vi "RT Main.vi"() -> ()   [LabVIEW 2025]
doc: "The myRIO Custom FPGA Project template acquires button data from the onboard button and displays the button value on a Boolean indicator. The SYS.RDY indicator shows the FPGA status."
uses:
  <vilib>/rvi/interface/nirviOpenFPGA/nirviOpenFPGA.xnode
  <vilib>/rvi/interface/nirviCloseFPGA/nirviCloseFPGA.xnode
  <vilib>/rvi/interface/nirviMethod/nirviMethod.xnode
  <vilib>/FPGAPlugInAG/Dynamic/niLvFpga_Run_Dynamic.vi
  SoC IP Library/SoC IP Library.lvlib
  SoC IP Library/Controls/Image Size.ctl
  <vilib>/vision/driver/NI_Vision_Acquisition_Software.lvlib
  <vilib>/userDefined/High Color/IMAQdx.ctl
  <vilib>/FPGAPlugInAG/Dynamic/niLvFpga_Reset_Dynamic.vi
  <vilib>/FPGAPlugInAG/Dynamic/niLvFpga_Close_Dynamic.vi
  FPGA Bitfiles/Final/FPGA_3x3_160MHz.lvbitx
  <vilib>/FPGAPlugInAG/myRIO-1900/niLvFpga_Open_myRIO-1900.vi
  <vilib>/rvi/interface/common/dynamic/niFpgaDynamicAddResources.vi
  FPGA Main 7-7 (Container).vi
  <vilib>/rvi/interface/RandomDataEmulation/nirviRandomDataOpen.vi
  <vilib>/rvi/interface/common/niFpgaCacheSessionInfoDynamic.vi
panel:
  in  "Display?":bool=TRUE
  out "Image Out":T1(plugin-control)
  out "Image In":T1(plugin-control)
  in  "Live":bool=TRUE
  in  "Timeout":i32=-1
  out "FPS":u32
  out "error out":errorcluster
  in  "Stop":bool
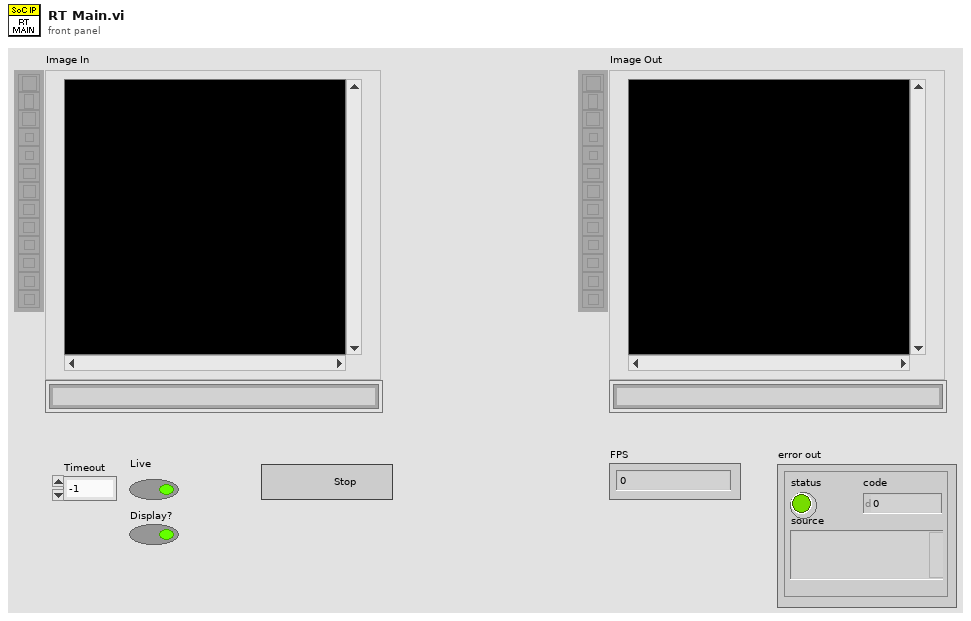
[diagram p1: front panel]
types:
  T1 = typedef "IMAQ Image.ctl" = refnum<image>
  T2 = typedef "IMAQdx.ctl" = refnum<k21>
  T3 = typedef "SoC IP Library.lvlib/Image Size.ctl" = cluster{"Rows (X)":u16, "Colums (Y)":u16}
  T4 = typedef "Image Type" = u32
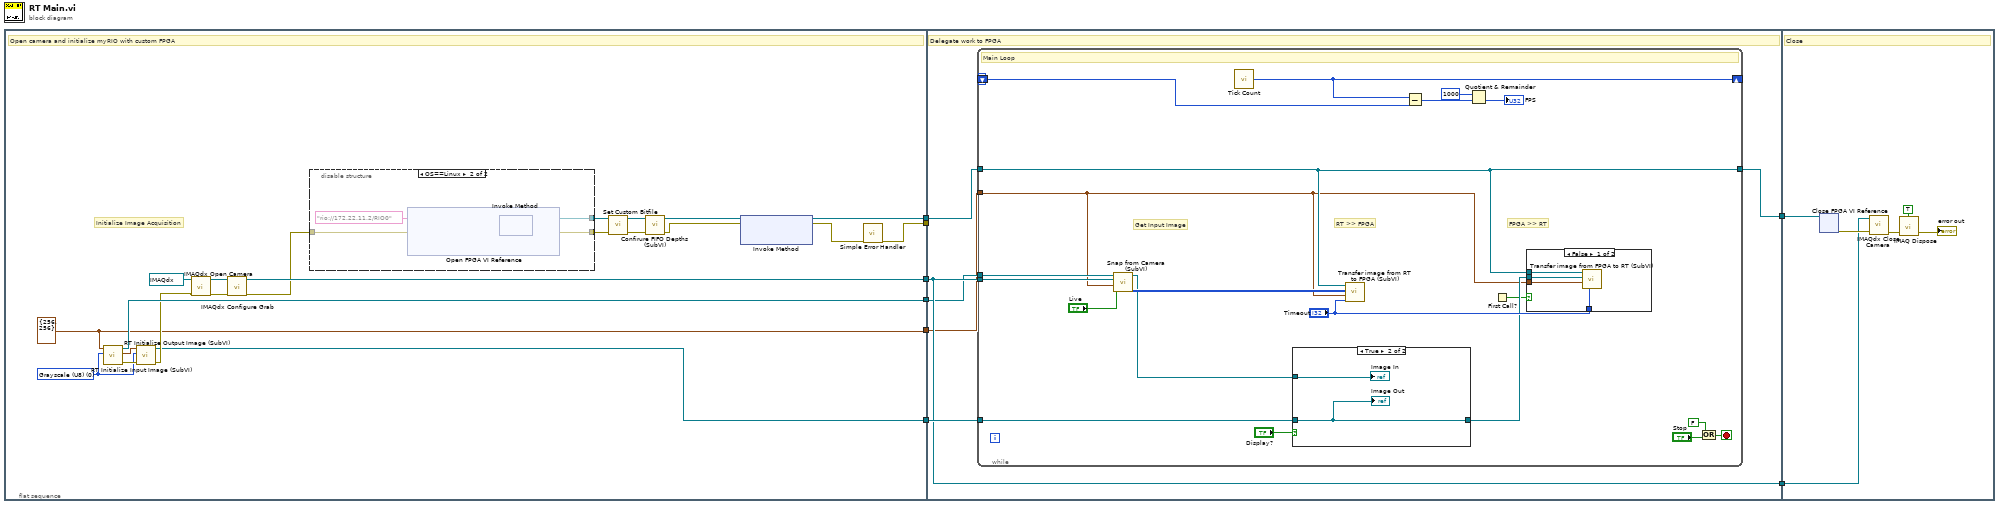
[diagram p0: block diagram]
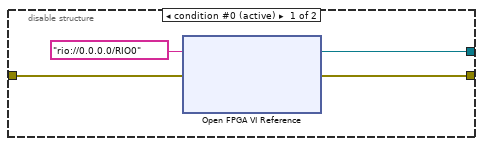
[diagram p2: hidden frame]
diagram:
  n1 = flat-sequence {
    tunnel: [w23] -> w8
    tunnel: [w28] -> w7
    tunnel: [w27] -> w6
    tunnel: [w17] -> w5
    tunnel: [w16] -> w3
    tunnel: [w15] -> w1
    tunnel: w8 -> [w45]
    tunnel: w7 -> [w43]
    tunnel: w6 -> [w42]
    tunnel: w5 -> [_]
    tunnel: [w43] -> w4
    tunnel: w3 -> [w44]
    tunnel: [w41] -> w2
    tunnel: w1 -> [w40]
    tunnel: w4 -> [w75]
    tunnel: w2 -> [w74]
    frame #0 {
      w15 = T3 {"Rows (X)"=256, "Colums (Y)"=256} ("Image Size")
      w24 = T4 0 items=["Grayscale (U8)", "Grayscale (I16)", "Grayscale (SGL)", "Complex (CSG)", "RGB (U32)", "HSL (U32)", "RGB (U64)", "Grayscale (U16)"] ("Image Type")
      # "Initialize Image Acquisition"
      # "Open camera and initialize myRIO with custom FPGA"
      n2 = call "RT Initialize Input Image (SubVI).vi"("Image Type"=w24, "Image Size In"=w15) -> ("error out"=w26:errorcluster, "Input Image Size Out"=w22:T3, "Input Image Out"=w27:T1)  [unwired: 7 in]
      n3 = call "RT Initialize Output Image (SubVI).vi"("error in (no error)"=w26, "Image Type"=w24, "Image Size In"=w22) -> ("error out"=w25:errorcluster, "Output Image Out"=w23:T1)  [unwired: 7 in]
      n4 = call <vilib>:"IMAQdx Open Camera.vi"("error in"=w25, "Session In"=T2 "cam0") -> ("error out"=w10:errorcluster, "Session Out"=w9:T2)  [unwired: 8 in]
      n5 = call <vilib>:"IMAQdx Configure Grab.vi"("error in"=w10, "Session In"=w9) -> ("error out"=w21:errorcluster, "Session Out"=w28:T2)  [unwired: 8 in]
      n6 = disable-structure shown="OS==Linux" {
        disable-tunnel: [w32 w36] -> w29
        disable-tunnel: [w30 w37] -> w13
        disable-tunnel: w21 -> [w31 w38]
        frame condition #0 (active) {
          n7 = xnode "Open FPGA VI Reference"("error in"=w31, "resource name"=tag "rio://0.0.0.0/RIO0") -> ("FPGA VI Reference Out"=w30:refnum<k20>, "error out"=w32:errorcluster)
        }
        frame condition #1 {
          n8 = xnode "Open FPGA VI Reference"("error in"=w38, "resource name"=tag "rio://172.22.11.2/RIO0") -> ("FPGA VI Reference Out"=w35:refnum<k20>, "error out"=w34:errorcluster)
          n9 = xnode "Invoke Method"("FPGA VI Reference In"=w35, "error in"=w34) -> ("FPGA VI Reference Out"=w37:refnum<k20>, "error out"=w36:errorcluster)
        }
      }
      n10 = call <vilib>:"Set Custom Bitfile.vi"("error in (no error)"=w29, "Custom FPGA Reference In"=w13) -> ("error out"=w19:errorcluster, "Custom FPGA Reference Out"=w12:refnum<k20>)  [unwired: 8 in]
      n11 = call "Confirure FIFO Depths (SubVI).vi"("error in (no error)"=w19, "Refnum in"=w12) -> ("error out"=w18:errorcluster, "Refnum out"=w14:refnum<k20>)  [unwired: 4 in, 4 out]
      n12 = xnode "Invoke Method"("FPGA VI Reference In"=w14, "error in"=w18) -> ("FPGA VI Reference Out"=w16:refnum<k20>, "error out"=w20:errorcluster)  [unwired: 1 in]
      n13 = call <vilib>:"Simple Error Handler.vi"("error in (no error)"=w20) -> ("error out"=w17:errorcluster)  [unwired: 4 in, 4 out]
    }
    frame #1 {
      # "Delegate work to FPGA"
      n14 = while {
        shift-right: [w64] -> _
        shift-left: u32 0 ("Tick Count(mSec)") -> [w63]
        tunnel: w44 -> [w56]
        tunnel: w43 -> [w62]
        tunnel: w45 -> [w55]
        tunnel: w42 -> [w61]
        tunnel: [w56] -> w41
        tunnel: w40 -> [w50]
        stop <- w65 stop-if-true
        # "FPGA >> RT"
        # "RT >> FPGA"
        # "Get Input Image"
        # "Main Loop"
        n15 = call "Snap from Camera (SubVI).vi"("Live"="Live", "Image Size in"=w50, "Session In"=w62, "Image in"=w61) -> ("Image Pixels (U8)"=w57:u8[][], "Image out"=w54:T1)  [unwired: 3 in, 3 out]
        n16 = call "Tick Count"() -> ("Tick Count(mSec)"=w64:u32)
        n17 = case shown="True" "Display?" {
          tunnel: w55 -> [w71 w73]
          tunnel: w54 -> [_ w72]
          tunnel: [w71 w73] -> w53
          frame False {
          }
          frame True {
            "Image In" <- w72
            "Image Out" <- w73
          }
        }
        n18 = call "Transfer image from RT to FPGA (SubVI).vi"("Timeout"="Timeout", "Image Size in"=w50, "Image Pixels (U8)"=w57, "FPGA Refnum in"=w56) -> ()  [unwired: 6 in, 2 out]
        n19 = Subtract(x=w64, y=w63) -> (x-y=w48:u32)
        n20 = Quotient & Remainder(x=u32 1000, y=w48) -> (floor(x/y)=→"FPS":u32)  [unwired: 1 out]
        n21 = First Call?() -> (First Call?: T/F=w51:bool)
        n22 = case shown="False" w51 {
          tunnel: "Timeout" -> [w70 _]
          tunnel: w56 -> [w69 _]
          tunnel: w53 -> [w68 _]
          tunnel: w50 -> [w67 _]
          frame False {
            n23 = call "Transfer image from FPGA to RT (SubVI).vi"("Timeout (ms)"=w70, "Image Size in"=w67, "Image In"=w68, "Refnum in"=w69) -> ()  [unwired: 5 in, 3 out]
          }
          frame True {
          }
        }
        n24 = Or(x=FALSE, y="Stop") -> (x .or. y?=w65:bool)
      }
    }
    frame #2 {
      # "Close"
      n25 = xnode "Close FPGA VI Reference"("FPGA VI Reference In"=w74) -> ("error out"=w77:errorcluster)  [unwired: 1 in]
      n26 = call <vilib>:"IMAQdx Close Camera.vi"("error in"=w77, "Session In"=w75) -> ("error out"=w76:errorcluster)  [unwired: 9 in]
      n27 = call "IMAQ Dispose"("All Images? (No)"=TRUE, "error in (no error)"=w76) -> ("error out"=→"error out":errorcluster)  [unwired: 4 in]
    }
  }
